vi "Periodic Tasks.vi"(8 "error in (no error)":errorcluster) -> ()   [LabVIEW 2014]
doc: "This VI runs in parallel to other tasks. It can contain as many user-defined periodic loops as you need. These can carry out PID or other sorts of timed response."
uses:
  <vilib>/Rock Robotics/SystemInterfaces/Utilities/FPGA_UtilitiesLED Source.ctl
  <vilib>/Rock Robotics/SystemInterfaces/Utilities/FPGA_UtilitiesLED State.ctl
  <vilib>/Rock Robotics/WPI/Relay/WPI_RelayValue.ctl
  <vilib>/Rock Robotics/WPI/DriverStation/WPI_DriverStationRobotMode2.ctl
  Robot Global Data.vi
  Robot Global ref.vi
  Events.vi
  <vilib>/ptbypt/NI_PtbyPt.lvlib
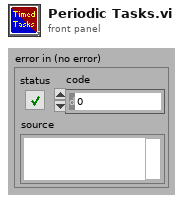
[diagram p1: front panel]
types:
  T1 = typedef "FPGA_UtilitiesLED State.ctl" = enum16{"Off", "On", "Toggle"}
  T2 = typedef "FPGA_UtilitiesLED Source.ctl" = enum16{"User LED", "FPGA LED"}
  T3 = typedef "Robot Global ref.ctl" = cluster{"Joysticks":cluster{"OpJoystickRef":T4, "DriveJoystickRef":T4, "DriveJoystickRef2":T4}, "Drive Motors Ref":cluster{"RobotDriveDevRef":T6}, "Ultrasonic":cluster{"AIDeviceRef":T14}, "Shifters":cluster{"SolenoidDevRef":T17}, "Gyro":cluster{"GyroDevRef":T20}, "Acquistion sensor":cluster{"HighDIO":T21, "Acquisition Bottom1":T21, "Acquisition Top":T21, "Acquisition Bottom2":T21}, "Motors":cluster{"AcqMotorRef":T7, "ShooterMotorRef":T7, "AcqshoulderControlDeviceRef":T7, "LatchControlDeviceRef":T7}, "Servos":cluster{"Winch Servo ":T23, "TrajectorycontrolDeviceRef":T23}, "Shooter Latch Sensors":cluster{"Shooter Latch Sensor Top":T21, "Shooter Latch Sensor Bottom":T21}, "Ring light relay":cluster{"RelayDevRef":T24}}
  T4 = typedef "WPI_JoystickDevRef.ctl" = cluster{"Device":T5}
  T5 = typedef "WPI_JoystickDeviceEnum.ctl" = enum16{"USB 0", "USB 1", "USB 2", "USB 3", "USB 4", "USB 5"}
  T6 = typedef "WPI_RobotDriveDevRef.ctl" = cluster{"DevStatus":errorcluster, "Motors[]":T7[], "Square Inputs":bool, "Max Output":dbl}
  T7 = typedef "WPI_MotorControlDeviceRef.ctl" = cluster{"DeviceStatus":errorcluster, "Type":enum16{"PWM", "CAN"}, "PWM":cluster{"Digital Module":T8, "PWM Channel":T9, "DeadBand":T10}, "CAN":cluster{"Device Number":u8, "Control Mode":T11, "Semaphore":T12, "Max Vout":dbl}, "Invert":bool, "TransformRef":T13, "InvTransformRef":T13}
  T8 = typedef "FPGA_TypedefDigitalModule.ctl" = enum16{"Digital Module 1", "Digital Module 2"}
  T9 = typedef "FPGA_DIOPWMChannel.ctl" = enum8{"PWM 1", "PWM 2", "PWM 3", "PWM 4", "PWM 5", "PWM 6", "PWM 7", "PWM 8", "PWM 9", "PWM 10", "Invalid"}
  T10 = typedef "WPI_PWMDeadband.ctl" = cluster{"Name":string, "maxPositivePwm":i32, "minPositivePwm":i32, "centerPwm":i32, "maxNegativePwm":i32, "minNegativePwm":i32, "angularRange":u16}
  T11 = typedef "WPI_CANJaguar_ControlMode.ctl" = enum8{"Percent VBus", "Current", "Speed", "Position", "Voltage"}
  T12 = typedef "Semaphore RefNum" = refnum<k1>
  T13 = typedef "WPI_PWMTransform_ConPane.ctl" = refnum<vi>
  T14 = typedef "WPI_AnalogChannelDevRef.ctl" = cluster{"DevStatus":errorcluster, "Analog Module":T15, "Analog Channel":T16}
  T15 = typedef "FPGA_TypedefAnalogModule.ctl" = enum16{"Analog Module 1", "Analog Module 2"}
  T16 = typedef "FPGA_AIChannel.ctl" = enum8{"AI 1", "AI 2", "AI 3", "AI 4", "AI 5", "AI 6", "AI 7", "AI 8", "Invalid"}
  T17 = typedef "WPI_SolenoidDevRef.ctl" = cluster{"DevStatus":errorcluster, "Solenoid Module":T18, "Forward Solenoid Channel":T19, "Reverse Solenoid Channel":T19}
  T18 = typedef "FPGA_TypedefSolenoidModule.ctl" = enum16{"Solenoid Module 1", "Solenoid Module 2"}
  T19 = typedef "WPI_SolenoidChannel.ctl" = enum8{"Solenoid 1", "Solenoid 2", "Solenoid 3", "Solenoid 4", "Solenoid 5", "Solenoid 6", "Solenoid 7", "Solenoid 8", "Invalid"}
  T20 = typedef "WPI_GyroDevRef.ctl" = cluster{"DevStatus":errorcluster, "Analog Module":T15, "Analog Channel":T16, "Offset":dbl, "Gain (VoltsPerDegree/Second)":dbl}
  T21 = typedef "WPI_DigitalInputDevRef.ctl" = cluster{"DevStatus":errorcluster, "DIO Channel":T22, "Digital Module":T8}
  T22 = typedef "FPGA_DIOChannel.ctl" = enum8{"DIO 1", "DIO 2", "DIO 3", "DIO 4", "DIO 5", "DIO 6", "DIO 7", "DIO 8", "DIO 9", "DIO 10", "DIO 11", "DIO 12", "DIO 13", "DIO 14", "Invalid"}
  T23 = typedef "WPI_ServoDeviceRef.ctl" = cluster{"DeviceStatus":errorcluster, "Digital Module":T8, "PWM Channel":T9, "DeadBand":T10}
  T24 = typedef "WPI_RelayDevRef.ctl" = cluster{"DevStatus":errorcluster, "Relay Channel":T25, "Digital Module":T8, "Relay Direction":T26}
  T25 = typedef "FPGA_DIORelayChannel.ctl" = enum8{"Relay 1", "Relay 2", "Relay 3", "Relay 4", "Relay 5", "Relay 6", "Relay 7", "Relay 8", "Invalid"}
  T26 = typedef "WPI_RelayDirection.ctl" = enum16{"Both directions", "Forward only", "Reverse only"}
  T27 = cluster{"Shooter Latch Sensor Top":T21, "Shooter Latch Sensor Bottom":T21}
  T28 = typedef "WPI_DriverStationRobotMode2.ctl" = enum16{"Autonomous Disabled", "Autonomous Enabled", "Teleop Disabled", "Teleop Enabled", "Disconnected", "Finish", "Test Disabled", "Test Enabled"}
  T29 = typedef "WPI_RelayValue.ctl" = enum16{"Off", "On", "Forward", "Reverse"}
  T30 = cluster{"Translate":dbl, "Y-Axis (Backward Speed)":dbl, "Rotate":dbl, "Tank right side":dbl, "axis 5":dbl, "axis 6":dbl, "Use gyro":bool, "Exponential\ndrive":bool, "Ring light":bool, "PID rotation":bool, "PID Gain":dbl}
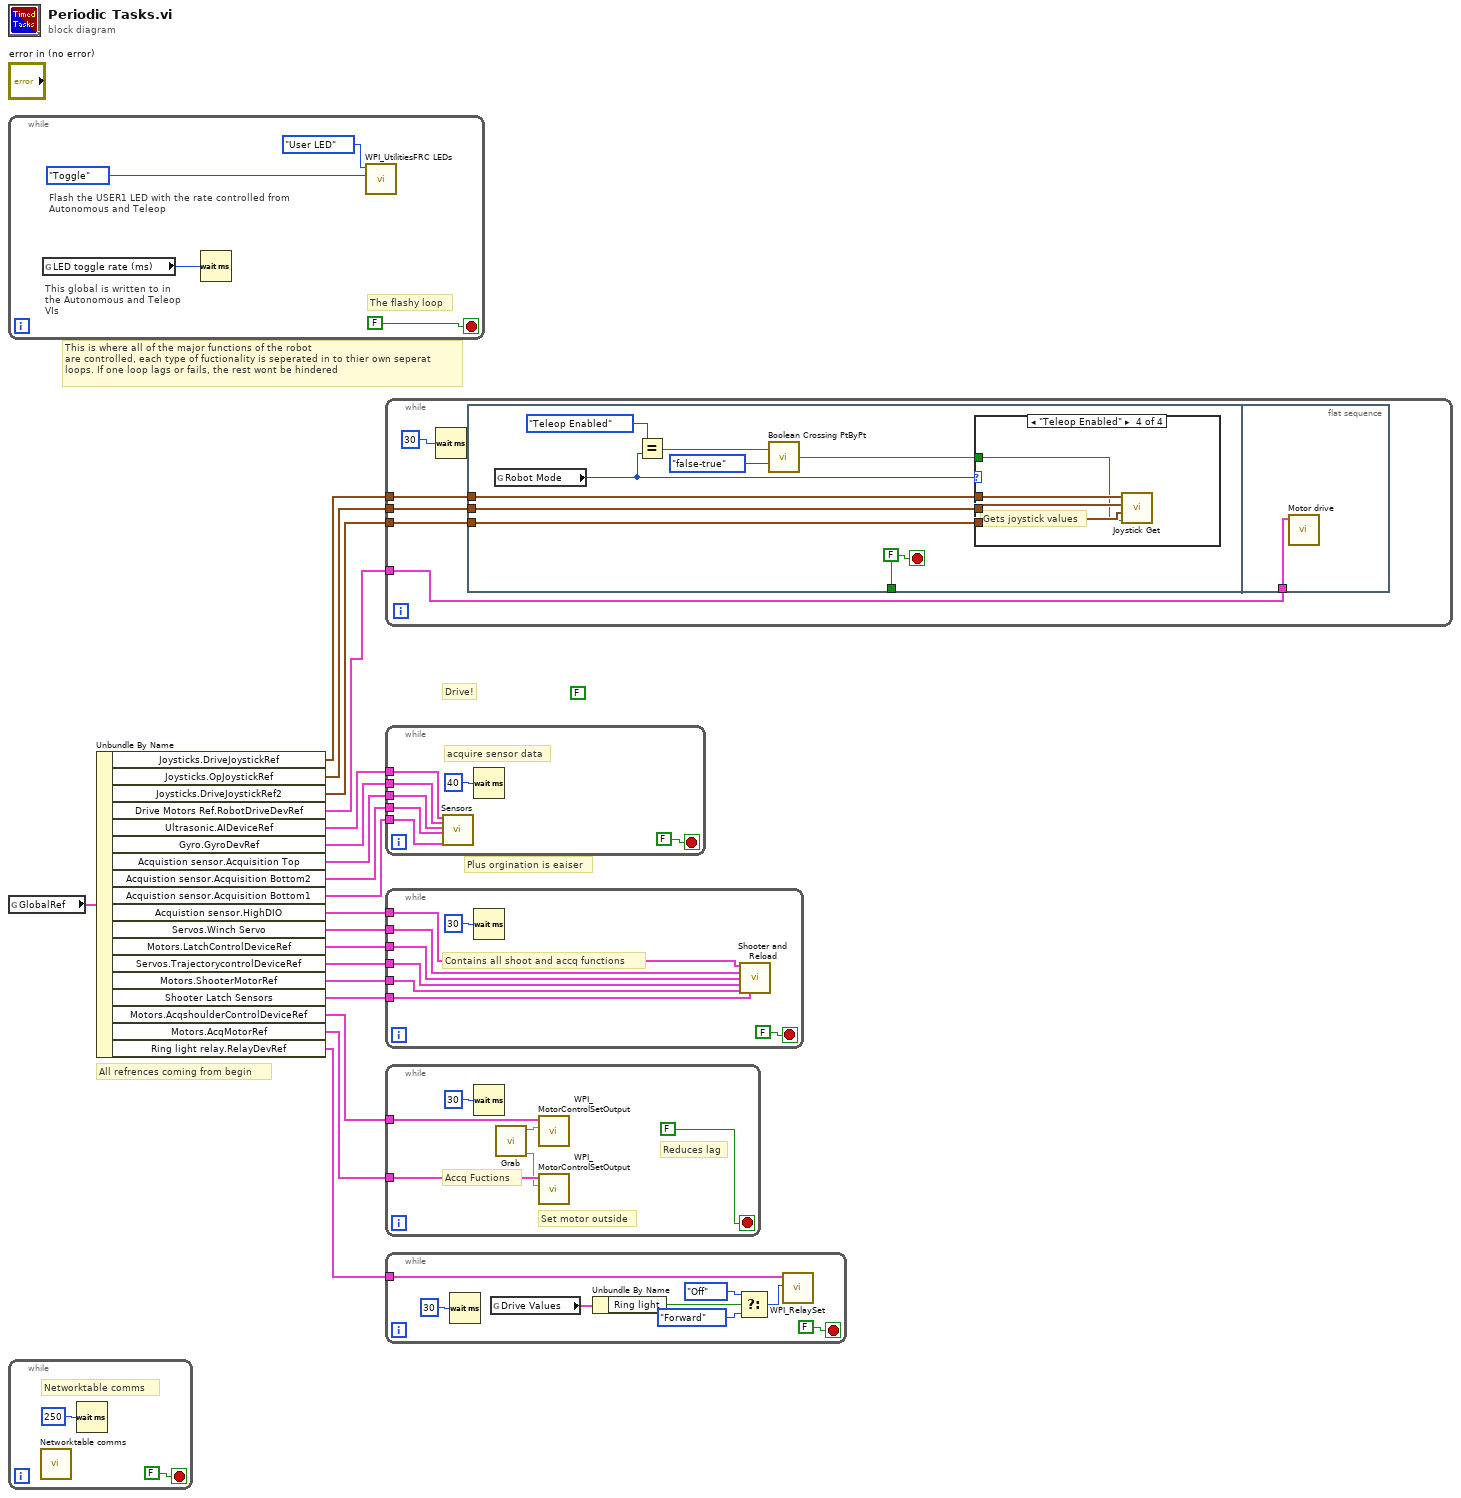
[diagram p0: block diagram]
diagram:
  (unwired) FALSE
  # "Drive!"
  # "Plus orgination is eaiser"
  # "This is where all of the major functions of the robot\nare controlled, each type of fuctionality is seperated in to thier own seperat \nloops. If one loop lags or fails, the rest wont be hindered"
  # "All refrences coming from begin"
  n1 = while {
    stop <- FALSE stop-if-true
    # "The flashy loop"
    # "This global is written to in the Autonomous and Teleop VIs"
    # "Flash the USER1 LED with the rate controlled from Autonomous and Teleop"
    n2 = global read "Robot Global Data.vi" "LED toggle rate (ms)"() -> (w20:u32)
    n3 = Wait (ms)(milliseconds to wait=w20) -> ()  [unwired: 1 out]
    n4 = call <vilib>:"WPI_UtilitiesFRC LEDs.vi"("State"=FPGA_UtilitiesLED_State."Toggle", "LED Type"=FPGA_UtilitiesLED_Source."User LED") -> ()  [unwired: 1 in, 9 out]
  }
  n5 = global read "Robot Global ref.vi" "GlobalRef"() -> (w19:T3)
  n6 = while {
    stop <- FALSE stop-if-true
    # "Networktable comms"
    n7 = call "Networktable comms.vi"() -> ()  [unwired: 12 in]
    n8 = Wait (ms)(milliseconds to wait=u32 250) -> ()  [unwired: 1 out]
  }
  n9 = Unbundle By Name(w19) -> ("Joysticks.DriveJoystickRef"=w16:T4, "Joysticks.OpJoystickRef"=w17:T4, "Joysticks.DriveJoystickRef2"=w18:T4, "Drive Motors Ref.RobotDriveDevRef"=w1:T6, "Ultrasonic.AIDeviceRef"=w8:T14, "Gyro.GyroDevRef"=w15:T20, "Acquistion sensor.Acquisition Top"=w14:T21, "Acquistion sensor.Acquisition Bottom2"=w2:T21, "Acquistion sensor.Acquisition Bottom1"=w9:T21, "Acquistion sensor.HighDIO"=w13:T21, "Servos.Winch Servo"=w10:T23, "Motors.LatchControlDeviceRef"=w7:T7, "Servos.TrajectorycontrolDeviceRef"=w4:T23, "Motors.ShooterMotorRef"=w6:T7, "Shooter Latch Sensors"=w5:T27, "Motors.AcqshoulderControlDeviceRef"=w12:T7, "Motors.AcqMotorRef"=w11:T7, "Ring light relay.RelayDevRef"=w3:T24)
  n10 = while {
    tunnel: w18 -> [w28]
    tunnel: w17 -> [w29]
    tunnel: w16 -> [w30]
    tunnel: w1 -> [w26]
    stop <- w31 stop-if-true
    n11 = Wait (ms)(milliseconds to wait=u32 30) -> ()  [unwired: 1 out]
    n12 = flat-sequence {
      tunnel: [FALSE] -> w31
      tunnel: w30 -> [w39]
      tunnel: w29 -> [w38]
      tunnel: w28 -> [w37]
      tunnel: w26 -> [w45]
      frame #0 {
        n13 = global read "Robot Global Data.vi" "Robot Mode"() -> (w36:T28)
        n14 = Equal?(x=WPI_DriverStationRobotMode2."Teleop Enabled", y=w36) -> (x = y?=w33:bool)
        n15 = call <vilib>:"Boolean Crossing PtByPt.vi"("direction"=enum16{"either", "false-true", "true-false"}."false-true", "input"=w33) -> ("crossing"=w32:bool)  [unwired: 1 in]
        n16 = case shown="\"Teleop Enabled\"" w36 {
          tunnel: w39 -> [_ _ _ w44]
          tunnel: w38 -> [_ _ _ w43]
          tunnel: w37 -> [_ _ _ w42]
          tunnel: w32 -> [_ _ _ w41]
          frame "Autonomous Disabled", Default {
          }
          frame "Autonomous Enabled" {
          }
          frame "Teleop Disabled" {
          }
          frame "Teleop Enabled" {
            # "Gets joystick values"
            n17 = call "Joystick Get.vi"("reset"=w41, "JoystickRefDrive 2"=w42, "JoystickRefOp"=w43, "JoystickRefDrive"=w44) -> ()  [unwired: 8 in]
          }
        }
      }
      frame #1 {
        n18 = call "Motor drive.vi"("RobotDriveDevRef"=w45) -> ()  [unwired: 10 in, 1 out]
      }
    }
  }
  n19 = while {
    tunnel: w15 -> [w50]
    tunnel: w14 -> [w49]
    tunnel: w9 -> [w48]
    tunnel: w8 -> [w47]
    tunnel: w2 -> [w46]
    stop <- FALSE stop-if-true
    # "acquire sensor data"
    n20 = call "Sensors.vi"("AIDeviceRef"=w47, "GyroDevRef"=w50, "Aquisition Sensor"=w49, "BottomAquistion 2"=w46, "BottomAquistion"=w48) -> ()  [unwired: 15 in]
    n21 = Wait (ms)(milliseconds to wait=u32 40) -> ()  [unwired: 1 out]
  }
  n22 = while {
    tunnel: w13 -> [w58]
    tunnel: w6 -> [w57]
    tunnel: w10 -> [w56]
    tunnel: w7 -> [w55]
    tunnel: w5 -> [w53]
    tunnel: w4 -> [w54]
    stop <- FALSE stop-if-true
    # "Contains all shoot and accq functions"
    n23 = Wait (ms)(milliseconds to wait=u32 30) -> ()  [unwired: 1 out]
    n24 = call "Shooter and Reload.vi"("Shooter at bottom limit"=w58, "Winch Shifter Servo"=w56, "LatchControlDevRef"=w55, "ServoDeviceRef"=w54, "ShooterWinchRef"=w57, "Shooter Latch Sensors"=w53) -> ()  [unwired: 10 in]
  }
  n25 = while {
    tunnel: w12 -> [w63]
    tunnel: w11 -> [w64]
    stop <- FALSE stop-if-true
    # "Reduces lag"
    # "Set motor outside"
    # "Accq Fuctions"
    n26 = Wait (ms)(milliseconds to wait=u32 30) -> ()  [unwired: 1 out]
    n27 = call "Grab.vi"() -> ("rollers"=w61:dbl, "shoulder"=w62:dbl)  [unwired: 8 in]
    n28 = call <vilib>:"WPI_MotorControlSetOutput.vi"("Output"=w62, "MotorControlDevRef"=w63) -> ()  [unwired: 7 in, 3 out]
    n29 = call <vilib>:"WPI_MotorControlSetOutput.vi"("Output"=w61, "MotorControlDevRef"=w64) -> ()  [unwired: 7 in, 3 out]
  }
  n30 = while {
    tunnel: w3 -> [w69]
    stop <- FALSE stop-if-true
    n31 = Wait (ms)(milliseconds to wait=u32 30) -> ()  [unwired: 1 out]
    n32 = global read "Events.vi" "Drive Values"() -> (w71:T30)
    n33 = Unbundle By Name(w71) -> ("Ring light"=w70:bool)
    n34 = Select(t=WPI_RelayValue."Off" ("RelayValue"), s=w70, f=WPI_RelayValue."Forward") -> (s? t:f=w73:T29)
    n35 = call <vilib>:"WPI_RelaySet.vi"("RelayValue"=w73, "RelayDevRef"=w69) -> ()  [unwired: 8 in, 2 out]
  }
